vi "setLimitsPolicy.vi"(11 "Device in":refnum<k24>) -> (3 "Device out":refnum<k24>)   [LabVIEW 2014]
doc: "André Romero - 2019\nandretec@ifsc.usp.br"
uses:
  C:/user-Lab/AndreTec/GITs/andretec/Thorlabs-Vector-Move/kinesisTec/Kinesis/Thorlabs.MotionControl.TCube.DCServoCLI.dll
  kinesisTec/Kinesis/Thorlabs.MotionControl.TCube.DCServoCLI.dll
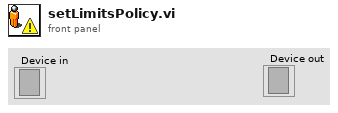
[diagram p1: front panel]
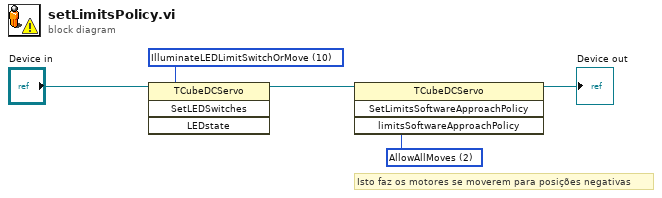
[diagram p0: block diagram]
diagram:
  w4 = i16 2 items=["DisallowIllegalMoves", "AllowPartialMoves", "AllowAllMoves"] ("limitsSoftwareApproachPolicy")
  w3 = 10 items=["None"=0, "FlashLEDIdent"=1, "IlluminateLEDLimitSwitch"=2, "IlluminateLEDIdentOrLimitSwitch"=3, "IlluminateLEDMove"=8, "IlluminateLEDIdentOrMove"=9, "IlluminateLEDLimitSwitchOrMove"=10, "IlluminateLEDAny"=11] ("LEDstate")
  # "Isto faz os motores se moverem para posições negativas"
  n1 = invoke class="TCubeDCServo" method="SetLEDSwitches"(reference="Device in", "LEDstate"=w3) -> (reference out=w2:refnum<k24>)  [unwired: 2 in, 3 out]
  n2 = invoke class="TCubeDCServo" method="SetLimitsSoftwareApproachPolicy"(reference=w2, "limitsSoftwareApproachPolicy"=w4) -> (reference out=→"Device out":refnum<k24>)  [unwired: 2 in, 3 out]
